vi "Calculate Number of steps.vi"(0 "Measurement Configuration":T1={"Quick Power Down"=FALSE, "Pin Name"=[], "Source Mode"=[], "Start Value"=[], "Target Value"=[], "Compliance Limit"=[], "Sense Mode"=[], "Default Ramp Rate"=[], "Ramp Rate"=[], "Start Delay"=[], "Relative To"=[], "Transient Response"=[], "Data Capture"=FALSE, "Power line frequency"=1} {"Power line frequency" items=["50 Hz", "60 Hz"]; "Start Value" format="%#_6p"; "Transient Response" items=["Slow", "Normal", "Fast"]; "Sense Mode" items=["Local Sense", "Remote Sense"]; "Relative To" items=["Power sequence start", "Previous source start", "Previous source end"]; "Target Value" format="%#_6p"; "Source Mode" items=["DC Voltage", "DC Current"]; "Start Delay" format="%#_6p"; "Compliance Limit" format="%#_6p"; "Ramp Rate" format="%#_6p"}, 5 "Minimum Sequence Delta":dbl[](array[numeric]), 11 "error in (no error)":errorcluster) -> (3 "Unsupported Ramp?":bool[](array[boolean]), 4 "Default Ramp Rate?":bool[](array[boolean]), 6 "Actual Ramp Rate[]":dbl[](array[numeric]), 8 "Number of steps[]":i32[](array[numeric]), 10 "Sequnence Delta[]":dbl[](array[numeric]), 15 "error out":errorcluster)   [LabVIEW 2024, in "devicePowerSequencerCoreLogic.lvlib"]
uses:
  devicePowerSequencerCoreLogic.lvlib
  Measurement Configuration.ctl
  controls/Source Mode.ctl
  controls/Sense Mode.ctl
  controls/Relative To.ctl
  controls/Transient Response.ctl
  controls/Power line frequency.ctl
  Device Power Sequencer.lvlib
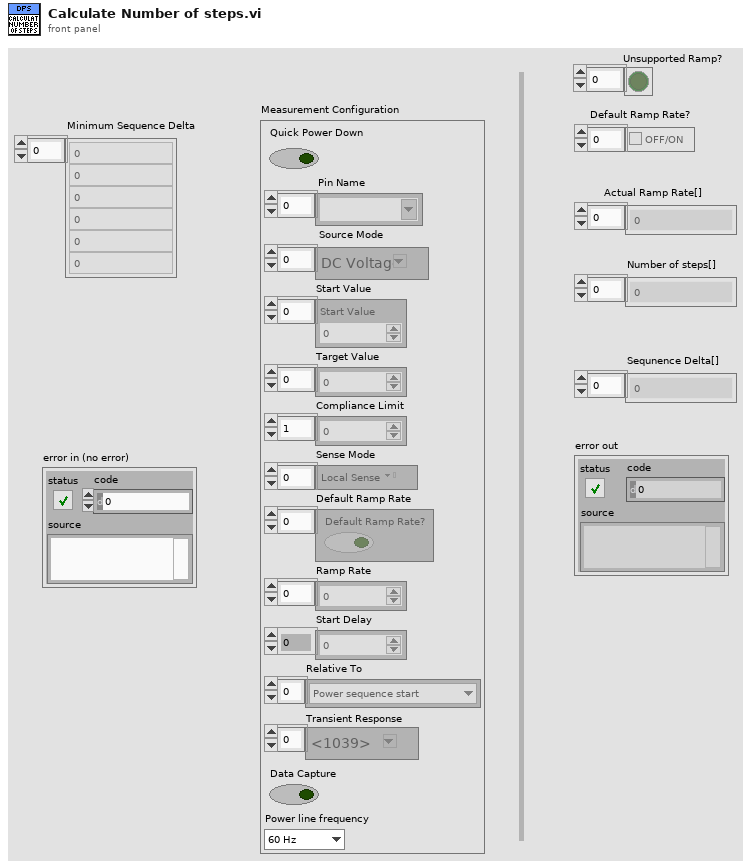
[diagram p1: front panel]
types:
  T1 = typedef "Device Power Sequencer.lvlib/Measurement Configuration.ctl" = cluster{"Quick Power Down":bool, "Pin Name":string[], "Source Mode":T2[], "Start Value":dbl[], "Target Value":dbl[], "Compliance Limit":dbl[], "Sense Mode":T3[], "Default Ramp Rate":bool[], "Ramp Rate":dbl[], "Start Delay":dbl[], "Relative To":T4[], "Transient Response":T5[], "Data Capture":bool, "Power line frequency":T6}
  T2 = typedef "Device Power Sequencer.lvlib/Source Mode.ctl" = i32
  T3 = typedef "Device Power Sequencer.lvlib/Sense Mode.ctl" = i32
  T4 = typedef "Device Power Sequencer.lvlib/Relative To.ctl" = u32
  T5 = typedef "Device Power Sequencer.lvlib/Transient Response.ctl" = i32
  T6 = typedef "Device Power Sequencer.lvlib/Power line frequency.ctl" = u32
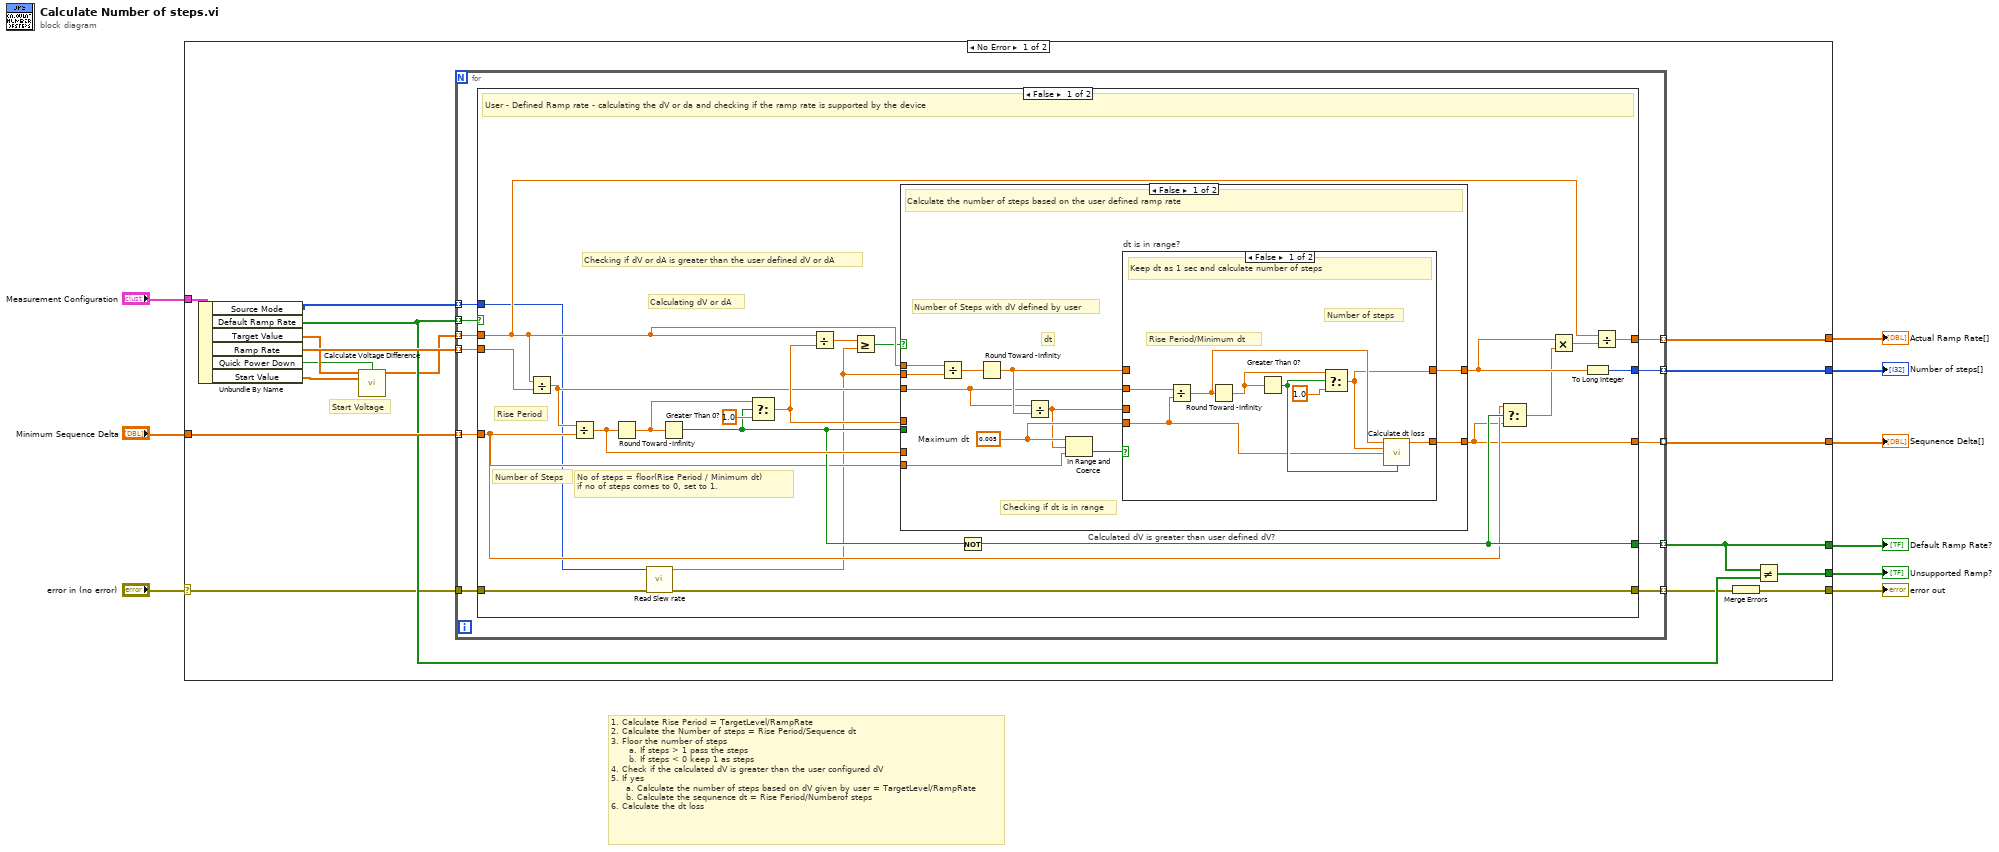
[diagram p0: block diagram]
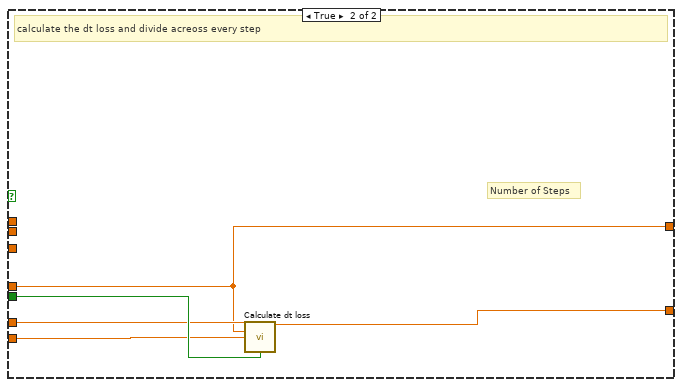
[diagram p3: hidden frame]
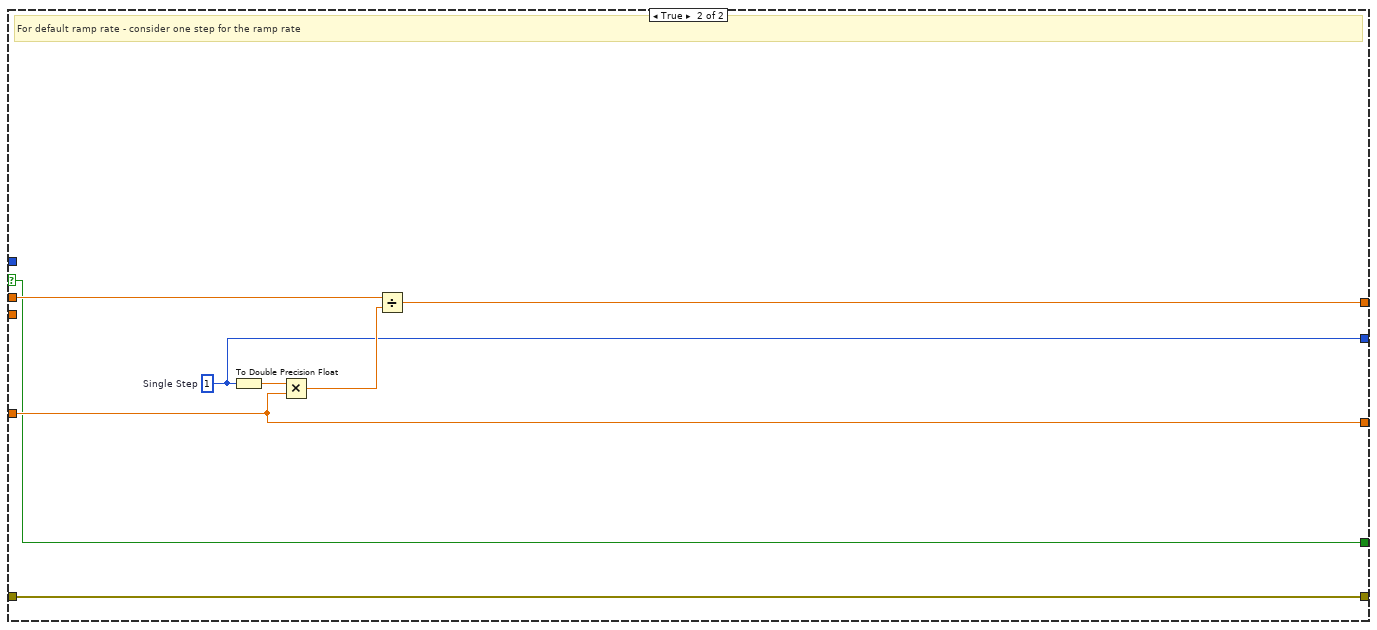
[diagram p4: hidden frame]
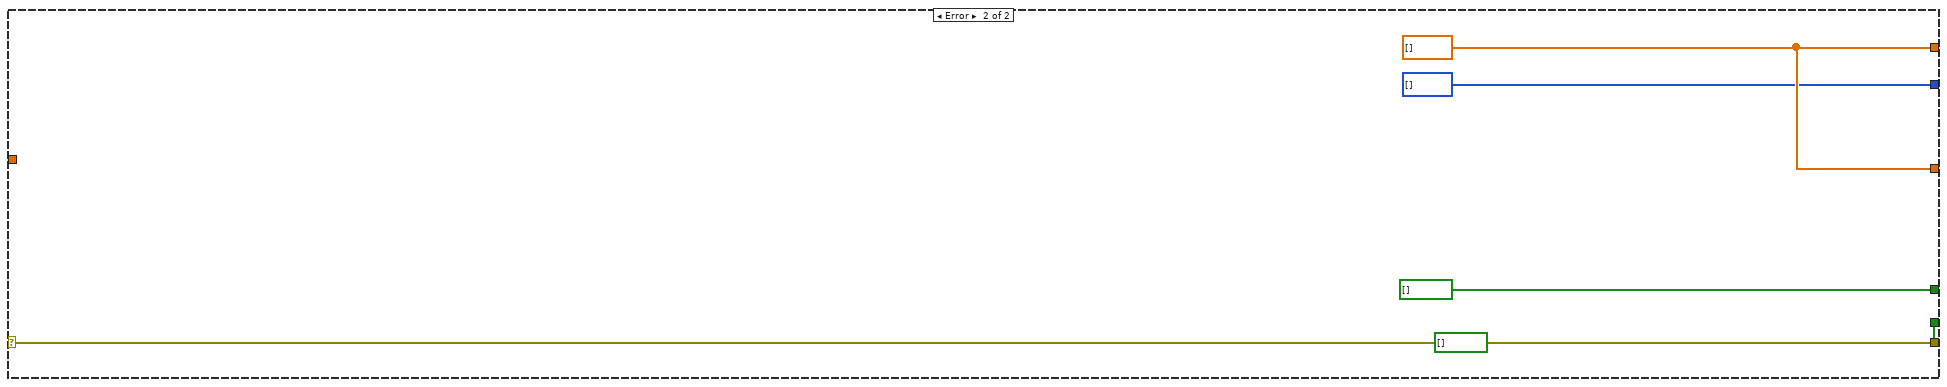
[diagram p5: hidden frame]
diagram:
  # "1. Calculate Rise Period = TargetLevel/RampRate\n2. Calculate the Number of steps = Rise Period/Sequence dt\n3. Floor the number of steps \n      a. If steps > 1 pass the steps\n      b. If steps < 0 keep 1 as steps\n4. Check if the calculated dV is greater than the user configured dV\n5. If yes \n     a. Calculate the number of steps based on dV given by user = TargetLevel/RampRate\n     b. Calculate the sequnence dt = Rise Period/Numberof steps\n6. Calculate the dt loss"
  n1 = case shown="No Error" "error in (no error)" {
    selector: "error in (no error)" -> [w12 w98]
    tunnel: "Measurement Configuration" -> [w26 _]
    tunnel: "Minimum Sequence Delta" -> [w25 _]
    tunnel: [w23 w97] -> w6
    tunnel: [w22 w97] -> w5
    tunnel: [w20 bool[] []] -> w3
    tunnel: [w10 w98] -> w4
    tunnel: [w21 i32[] []] -> w2
    tunnel: [w18 bool[] []] -> w1
    frame No Error {
      # "Start Voltage"
      n2 = Unbundle By Name(w26) -> ("Source Mode"=w13:T2[], "Default Ramp Rate"=w19:bool[], "Target Value"=w16:dbl[], "Ramp Rate"=w24:dbl[], "Quick Power Down"=w14:bool, "Start Value"=w15:dbl[])
      n3 = call "Calculate Voltage Difference.vi"("Target Value"=w16, "PowerUp?"=w14, "Start Value"=w15) -> ("Value  difference"=w17:dbl[])  [unwired: 12 in]
      n4 = for {
        tunnel: w25 -> [w34] mode=indexing
        tunnel: w19 -> [w37] mode=indexing
        tunnel: w17 -> [w36] mode=indexing
        tunnel: w24 -> [w35] mode=indexing
        tunnel: [w33] -> w23 mode=indexing
        tunnel: [w32] -> w22 mode=indexing
        tunnel: [w31] -> w21 mode=indexing
        tunnel: [w30] -> w20 mode=indexing
        tunnel: w13 -> [w29] mode=indexing
        tunnel: w12 -> [w28]
        tunnel: [w27] -> w11 mode=indexing
        n5 = case shown="False" w37 {
          selector: w37 -> [_ w87]
          tunnel: w36 -> [w51 w92]
          tunnel: w35 -> [w47 _]
          tunnel: w34 -> [w44 w88]
          tunnel: [w50 w90] -> w33
          tunnel: [w43 w88] -> w32
          tunnel: [w49 w89] -> w31
          tunnel: [w45 w87] -> w30
          tunnel: w29 -> [w40 _]
          tunnel: w28 -> [w41 w86]
          tunnel: [w38 w86] -> w27
          frame False {
            # "No of steps = floor(Rise Period / Minimum dt)\nif no of steps comes to 0, set to 1."
            # "Checking if dV or dA is greater than the user defined dV or dA"
            # "Calculating dV or dA"
            # "Number of Steps"
            # "Rise Period"
            # "User - Defined Ramp rate - calculating the dV or da and checking if the ramp rate is supported by the device"
            n6 = Divide(x=w51, y=w47) -> (x/y=w54:dbl)
            n7 = Divide(x=w54, y=w44) -> (x/y=w55:dbl)
            n8 = Round Toward -Infinity(1:w55) -> (0:w58:dbl)
            n9 = call "Read Slew rate.vi"("Source Mode"=w40, "error in (no error)"=w41) -> ("Min Change"=w39:dbl, "error out"=w38:errorcluster)  [unwired: 12 in]
            n10 = Greater Than 0?(x=w58) -> (x > 0?=w48:bool)
            n11 = Select(t=w58, s=w48, f=1.0) -> (s? t:f=w56:dbl)
            n12 = Divide(x=w51, y=w56) -> (x/y=w57:dbl)
            n13 = Greater Or Equal?(x=w57, y=w39) -> (x >= y?=w46:bool)
            n14 = case "Calculated dV is greater than user defined dV?" shown="False" w46 {
              tunnel: w48 -> [_ w85]
              tunnel: w56 -> [_ w81]
              tunnel: w55 -> [_ w82]
              tunnel: w44 -> [w67 w84]
              tunnel: [w63 w83] -> w43
              tunnel: w51 -> [w70 _]
              tunnel: w39 -> [w68 _]
              tunnel: w54 -> [w64 _]
              tunnel: [w61 w81] -> w53
              frame False {
                w65 = 0.005  # Maximum dt
                # "Checking if dt is in range"
                # "dt"
                # "Number of Steps with dV defined by user"
                # "Calculate the number of steps based on the user defined ramp rate"
                n15 = Divide(x=w70, y=w68) -> (x/y=w69:dbl)
                n16 = Round Toward -Infinity(1:w69) -> (0:w66:dbl)
                n17 = Divide(x=w64, y=w66) -> (x/y=w62:dbl)
                n18 = In Range and Coerce(upper limit=w65, x=w62, lower limit=w67) -> (In Range?=w60:bool)  [unwired: 1 out]
                n19 = case "dt is in range?" shown="False" w60 {
                  tunnel: [w71 w80] -> w61
                  tunnel: w66 -> [_ w80]
                  tunnel: w65 -> [w74 _]
                  tunnel: w64 -> [w78 _]
                  tunnel: [w73 w79] -> w63
                  tunnel: w62 -> [_ w79]
                  frame False {
                    # "Number of steps"
                    # "Rise Period/Minimum dt"
                    # "Keep dt as 1 sec and calculate number of steps"
                    n20 = Divide(x=w78, y=w74) -> (x/y=w72:dbl)
                    n21 = Round Toward -Infinity(1:w72) -> (0:w75:dbl)
                    n22 = Greater Than 0?(x=w75) -> (x > 0?=w76:bool)
                    n23 = Select(t=w75, s=w76, f=1.0) -> (s? t:f=w71:dbl)
                    n24 = call "Calculate dt loss.vi"("No. of Steps"=w72, "Floor(No.ofSteps)"=w71, "Minimum Sequence Delta (S)"=w74, "No. of steps is greater than 0?"=w76) -> ("Minimum Sequence Delta (S)"=w73:dbl)  [unwired: 11 in]
                  }
                  frame True {
                    # "Pass the Number of steps and\nMinimum sequence delta"
                  }
                }
              }
              frame True {
                # "Number of Steps"
                # "calculate the dt loss and divide acreoss every step"
                n25 = call "Calculate dt loss.vi"("No. of Steps"=w82, "Floor(No.ofSteps)"=w81, "Minimum Sequence Delta (S)"=w84, "No. of steps is greater than 0?"=w85) -> ("Minimum Sequence Delta (S)"=w83:dbl)  [unwired: 11 in]
              }
            }
            n26 = Not(x=w48) -> (.not. x?=w45:bool)
            n27 = Select(t=w44, s=w45, f=w43) -> (s? t:f=w42:dbl)
            n28 = Multiply(x=w53, y=w42) -> (x*y=w52:dbl)
            n29 = To Long Integer(number=w53) -> (32bit integer=w49:i32)
            n30 = Divide(x=w51, y=w52) -> (x/y=w50:dbl)
          }
          frame True {
            w89 = 1  # Single Step
            # "For default ramp rate - consider one step for the ramp rate"
            n31 = To Double Precision Float(number=w89) -> (double precision float=w93:dbl)
            n32 = Multiply(x=w93, y=w88) -> (x*y=w91:dbl)
            n33 = Divide(x=w92, y=w91) -> (x/y=w90:dbl)
          }
        }
      }
      n34 = Merge Errors(w11) -> (w10:errorcluster)
      n35 = Not Equal?(x=w20, y=w19) -> (x != y?=w18:bool[])
    }
    frame Error {
      w97 = dbl[] []
    }
  }
  "error out" <- w4
  "Sequnence Delta[]" <- w5
  "Number of steps[]" <- w2
  "Actual Ramp Rate[]" <- w6
  "Default Ramp Rate?" <- w3
  "Unsupported Ramp?" <- w1
